vi "Remove Key.vi"(8 "error in (no error)":errorcluster, 10 "Key":string, 11 "E2E editor node in":refnum<data-value>) -> (0 "error out":errorcluster, 3 "E2E editor node out":refnum<data-value>)   [LabVIEW 2015, in "E2E Tag Exchange editor node.lvclass"]
uses:
  E2E Tag Exchange editor node.lvclass
  module/configuration/E2E Tag Exchange configuration.lvclass
  <vilib>/NI/Configuration Framework/serializable configuration/NISE_CEF_serializable configuration.lvclass
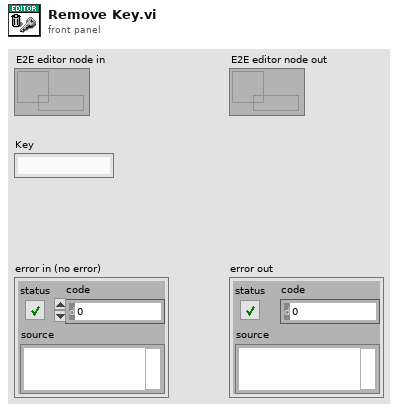
[diagram p1: front panel]
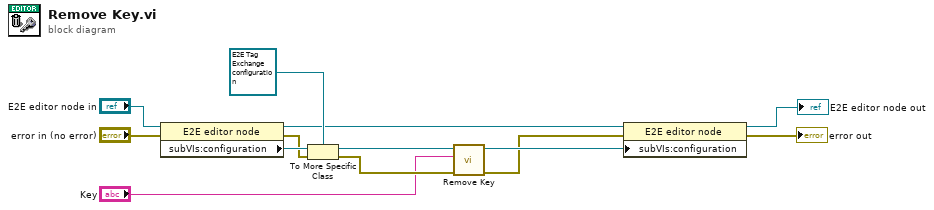
[diagram p0: block diagram]
diagram:
  n1 = property class="E2E editor node"(reference="E2E editor node in", error in="error in (no error)") -> (reference out=w8:refnum<data-value>, error out=w11:errorcluster, "subVIs:configuration"=w12:refnum<class "NISE_CEF_serializable configuration.lvclass">)
  n2 = To More Specific Class(target class=refnum<class "E2E Tag Exchange configuration.lvclass"> refnum ("E2E configuration"), reference=w12, error in=w11) -> (specific class reference=w4:refnum<class "E2E Tag Exchange configuration.lvclass">, error out=w5:errorcluster)
  n3 = call "Remove Key.vi"("error in"=w5, "Key"="Key", "E2E configuration in"=w4) -> ("error out"=w2:errorcluster, "E2E configuration out"=w3:refnum<class "E2E Tag Exchange configuration.lvclass">)  [unwired: 7 in]
  n4 = property class="E2E editor node"(reference=w8, error in=w2, "subVIs:configuration"=w3) -> (reference out=→"E2E editor node out":refnum<data-value>, error out=→"error out":errorcluster)
